vi "ROI entry-Create centered ROI.vi"(8 "error in (no error)":errorcluster, 11 "Coordinates":i32[](array[numeric])) -> (0 "error out":errorcluster, 1 "Do not generate ROI":bool, 3 "ROIs Info []":T1[](array[typedef]) {"FOV" min=1.0 max=10.0 step=1.0; "Frame Size" min=1.0 max=10.0 step=1.0; "Laser Power" min=1.0 max=10.0 step=0.10000000149011612; "Rel. Resolution" min=1.0 max=10.0 step=1.0; "POI Dwell time" min=1.0 max=10.0 step=0.10000000149011612; "Zoom" min=1.0 max=10.0 step=0.10000000149011612})   [LabVIEW 2020]
uses:
  Typedefs/ROI spec.ctl
  Typedefs/ROI ID Enum.ctl
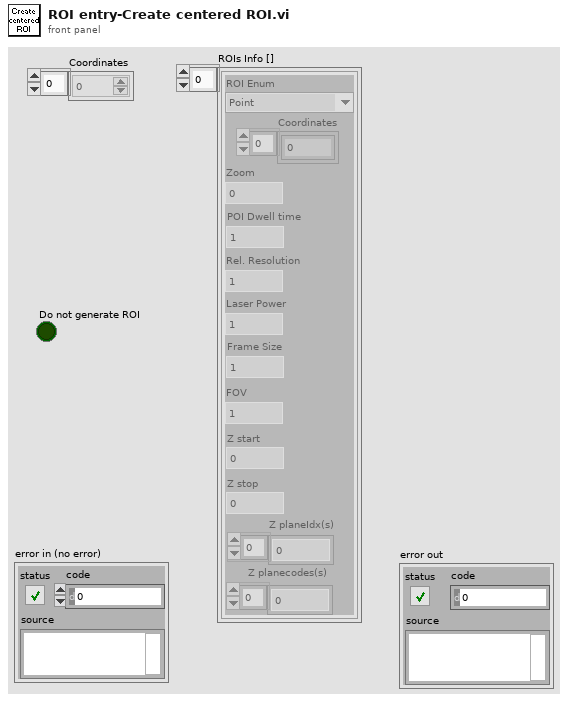
[diagram p1: front panel]
types:
  T1 = typedef "ROI spec.ctl" = cluster{"ROI Enum":T2, "Coordinates":i32[], "Zoom":dbl, "POI Dwell time":dbl, "Rel. Resolution":dbl, "Laser Power":dbl, "Frame Size":dbl, "FOV":dbl, "Z start":dbl, "Z stop":dbl, "Z planeIdx(s)":i32[], "Z planecodes(s)":u8[]}
  T2 = typedef "ROI ID Enum.ctl" = enum16{"Point", "MiniScan", "Comp. MiniScan", "Rectangle", "Comp. volume", "Arb. plane point", "None"}
  T3 = typedef "ROI Z-stack settings info.ctl" = cluster{"Zoom":dbl, "POI Dwell time":dbl, "Rel. Res":dbl, "Laser Power %":dbl, "Frame Size":dbl, "FOV":dbl}
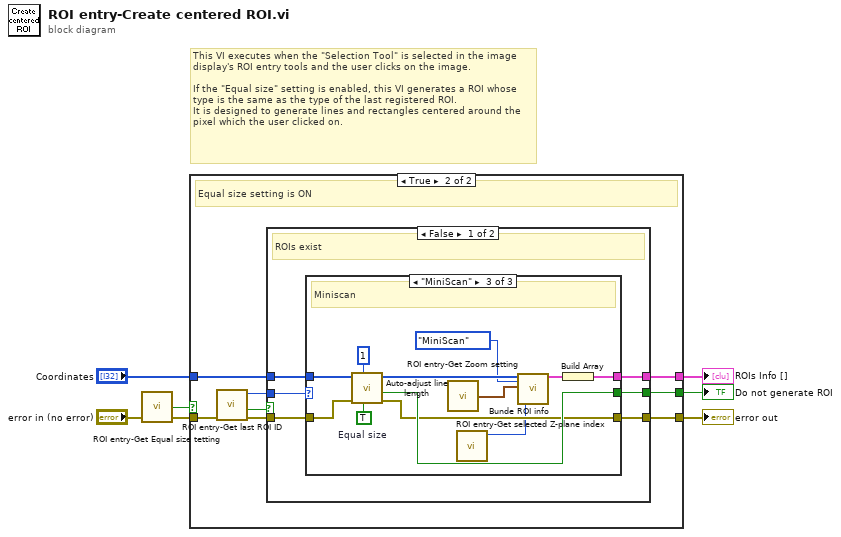
[diagram p0: block diagram]
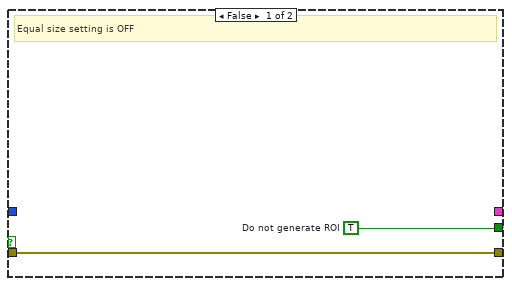
[diagram p2: hidden frame]
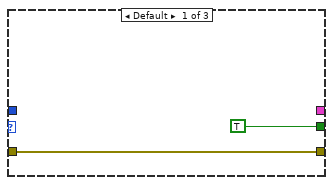
[diagram p3: hidden frame]
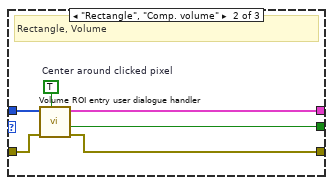
[diagram p4: hidden frame]
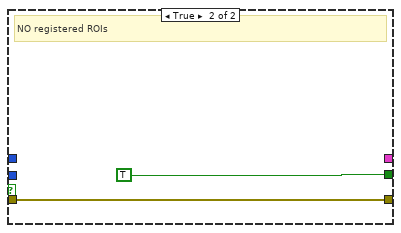
[diagram p5: hidden frame]
diagram:
  # "This VI executes when the \"Selection Tool\" is selected in the image display's ROI entry tools and the user clicks on the image.\n\nIf the \"Equal size\" setting is enabled, this VI generates a ROI whose type is the same as the type of the last registered ROI.\nIt is designed to generate lines and rectangles centered around the pixel which the user clicked on."
  n1 = call "ROI entry-Get Equal size tetting.vi"("error in (no error)"="error in (no error)") -> ("error out"=w6:errorcluster, "Equal size setting's value"=w4:bool)  [unwired: 3 in]
  n2 = case shown="True" w4 {
    tunnel: "Coordinates" -> [_ w17]
    tunnel: [w9 w16] -> w3
    tunnel: [w8 w15] -> w7
    tunnel: w6 -> [w8 w13]
    tunnel: [_ w10] -> w1
    frame False {
      w9 = TRUE  # Do not generate ROI
      # "Equal size setting is OFF"
    }
    frame True {
      # "Equal size setting is ON"
      n3 = call "ROI entry-Get last ROI ID.vi"("error in (no error)"=w13) -> ("error out"=w12:errorcluster, "NO ROI"=w11:bool, "ROI ID Enum"=w14:T2)  [unwired: 7 in, 1 out]
      n4 = case shown="False" w11 {
        tunnel: w17 -> [w23 _]
        tunnel: [w22 TRUE ("Do not generate ROI")] -> w16
        tunnel: [w21 w44] -> w15
        tunnel: w14 -> [w20 _]
        tunnel: w12 -> [w19 w44]
        tunnel: [w18 _] -> w10
        frame False {
          # "ROIs exist"
          n5 = case shown="\"MiniScan\"" w20 {
            tunnel: w23 -> [_ w31 w43]
            tunnel: [TRUE ("Do not generate ROI") w30 w35] -> w22
            tunnel: w19 -> [w24 w29 w40]
            tunnel: [w24 w28 w34] -> w21
            tunnel: [_ w26 w36] -> w18
            frame Default {
            }
            frame "Rectangle", "Comp. volume" {
              w27 = TRUE  # Center around clicked pixel
              # "Rectangle, Volume"
              n6 = call "Volume ROI entry user dialogue handler.vi"("Center around clicked pixel (F)"=w27, "error in (no error)"=w29, "New coordinates"=w31) -> ("error IO"=w28:errorcluster, "Cancelled"=w30:bool, "ROIs Info []"=w26:T1[])  [unwired: 6 in]
            }
            frame "MiniScan" {
              w41 = TRUE  # Equal size
              # "Miniscan"
              n7 = call "Auto-adjust line length.vi"("Equal size"=w41, "Current ROI Tool"=1, "error in (no error)"=w40, "New Coordinates"=w43) -> ("error out"=w34:errorcluster, "Do not generate ROI"=w35:bool, "Output coordinates"=w39:i32[])  [unwired: 5 in]
              n8 = call "ROI entry-Get Zoom setting.vi"() -> ("AOLZ Settings"=w32:T3)  [unwired: 7 in, 8 out]
              n9 = call "ROI entry-Get selected Z-plane index.vi"() -> ("Z-plane selector (index)"=w33:i32)  [unwired: 10 in, 1 out]
              n10 = call "Bunde ROI info.vi"("ROI Coordinates"=w39, "ROI Enum"=ROI_ID_Enum."MiniScan" ("ROI Type"), "Z stack Settings"=w32, "ZplaneIndex"=w33) -> ("ROI Info"=w37:T1)  [unwired: 15 in]
              n11 = Build Array(w37) -> (w36:T1[])
            }
          }
        }
        frame True {
          # "NO registered ROIs"
        }
      }
    }
  }
  "error out" <- w7
  "Do not generate ROI" <- w3
  "ROIs Info []" <- w1
